vi "testing format SEQLIST array.vi"(4 "Test Station? (f)":bool, 6 "User Information":T1, 11 "Results":T2[](array[typedef])) -> (3 "SEQLIST array":string)   [LabVIEW 2011]
uses:
  server/database/Sequences/Sequence Record.ctl
  server/database/Users/User Record.ctl
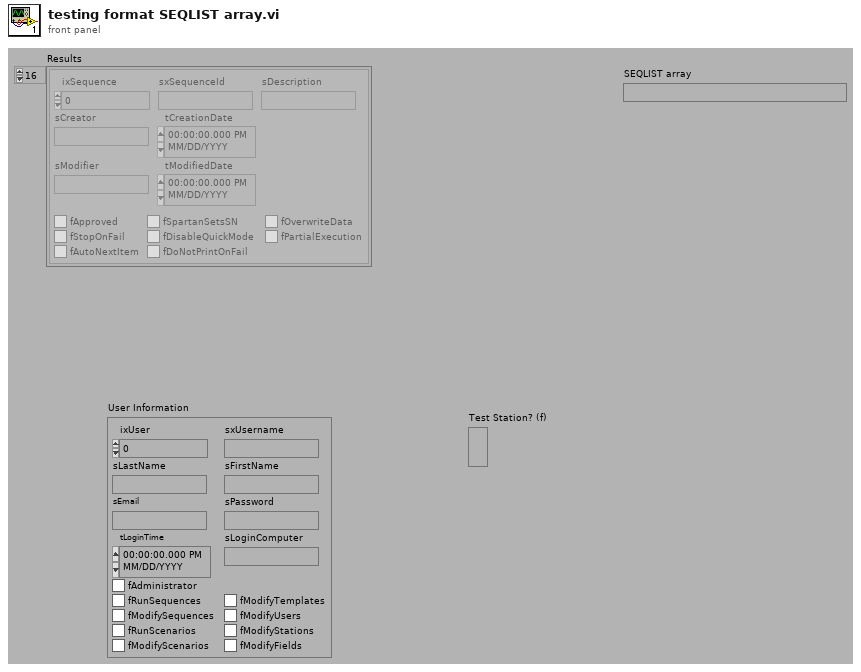
[diagram p1: front panel]
types:
  T1 = typedef "User Record.ctl" = cluster{"ixUser":i32, "sxUsername":string, "sLastName":string, "sFirstName":string, "sEmail":string, "sPassword":string, "tLoginTime":timestamp, "sLoginComputer":string, "fAdministrator":bool, "fRunSequences":bool, "fModifySequences":bool, "fRunScenarios":bool, "fModifyScenarios":bool, "fModifyTemplates":bool, "fModifyUsers":bool, "fModifyStations":bool, "fModifyFields":bool}
  T2 = typedef "Sequence Record.ctl" = cluster{"ixSequence":i32, "sxSequenceId":string, "sDescription":string, "sCreator":string, "tCreationDate":timestamp, "sModifier":string, "tModifiedDate":timestamp, "fApproved":bool, "fSpartanSetsSN":bool, "fOverwriteData":bool, "fStopOnFail":bool, "fDisableQuickMode":bool, "fPartialExecution":bool, "fAutoNextItem":bool, "fDoNotPrintOnFail":bool}
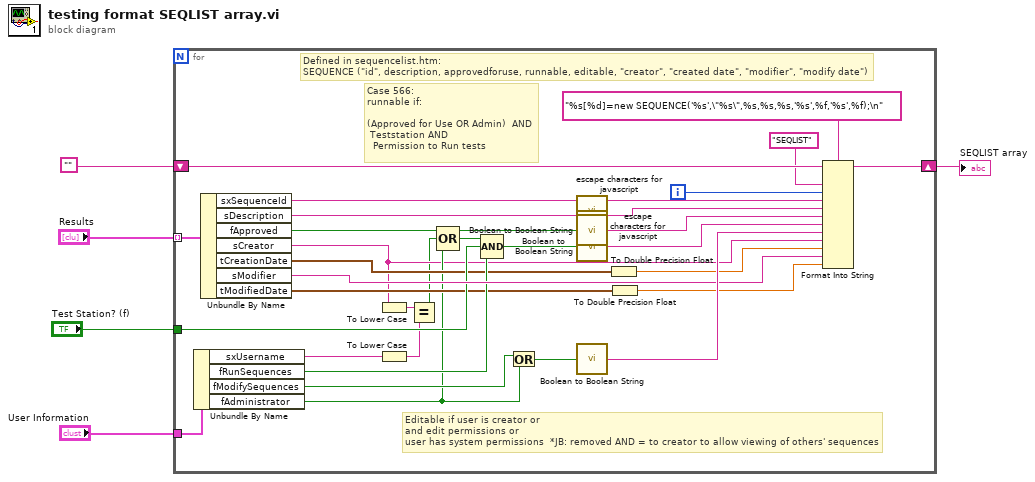
[diagram p0: block diagram]
diagram:
  n1 = for {
    tunnel: "Results" -> [w33] mode=indexing
    shift-right: [w34] -> w4
    shift-left: "" -> [w36]
    tunnel: "User Information" -> [w30]
    tunnel: "Test Station? (f)" -> [w23]
    i -> [w35]
    # "Case 566:\nrunnable if:\n\n(Approved for Use OR Admin)  AND\n Teststation AND\n  Permission to Run tests"
    # "Editable if user is creator or\nand edit permissions or\nuser has system permissions  *JB: removed AND = to creator to allow viewing of others' sequences"
    # "Defined in sequencelist.htm:\nSEQUENCE (\"id\", description, approvedforuse, runnable, editable, \"creator\", \"created date\", \"modifier\", \"modify date\")"
    n2 = Unbundle By Name(w30) -> ("sxUsername"=w10:string, "fRunSequences"=w22:bool, "fModifySequences"=w24:bool, "fAdministrator"=w12:bool)
    n3 = Unbundle By Name(w33) -> ("sxSequenceId"=w15:string, "sDescription"=w17:string, "fApproved"=w13:bool, "sCreator"=w9:string, "tCreationDate"=w21:timestamp, "sModifier"=w25:string, "tModifiedDate"=w19:timestamp)
    n4 = To Lower Case(string=w9) -> (all lower case string=w7:string)
    n5 = To Lower Case(string=w10) -> (all lower case string=w8:string)
    n6 = Equal?(x=w7, y=w8) -> (x = y?=w6:bool)
    n7 = Compound Arithmetic op=OR(w13, w6, w12) -> (w11:bool)
    n8 = Compound Arithmetic op=AND(w11, w23, w22) -> (w29:bool)
    n9 = Or(x=w24, y=w12) -> (x .or. y?=w26:bool)
    n10 = call "escape characters for javascript.vi"("String (\"\")"=w15) -> ("escaped String"=w14:string)  [unwired: 4 out]
    n11 = call "escape characters for javascript.vi"("String (\"\")"=w17) -> ("escaped String"=w16:string)  [unwired: 4 out]
    n12 = call "Boolean to Boolean String.vi"("Boolean"=w13) -> ("Boolean string"=w31:string)  [unwired: 1 in]
    n13 = call "Boolean to Boolean String.vi"("Boolean"=w29) -> ("Boolean string"=w28:string)  [unwired: 1 in]
    n14 = call "Boolean to Boolean String.vi"("Boolean"=w26) -> ("Boolean string"=w27:string)  [unwired: 1 in]
    n15 = To Double Precision Float(number=w21) -> (double precision float=w20:dbl)
    n16 = To Double Precision Float(number=w19) -> (double precision float=w18:dbl)
    n17 = Format Into String(format string="%s[%d]=new SEQUENCE('%s',\"%s\",%s,%s,%s,'%s',%f,'%s',%f);\n", initial string=w36, "SEQLIST", w35, w14, w16, w31, w28, w27, w9, w20, w25, w18) -> (resulting string=w34:string)  [unwired: 1 in, 1 out]
  }
  "SEQLIST array" <- w4
